vi "相关系数.vi"() -> ()   [LabVIEW 2018]
uses:
  <vilib>/gmath/NI_Gmath.lvlib
panel:
  in  "停止":bool
  out "r^2":dbl format="%.7g"
  out "correlation coefficient r":dbl caption="相关系数r" format="%.7g"
  in  "数组 2":dbl[](array[numeric])
  in  "数组":dbl[](array[numeric])
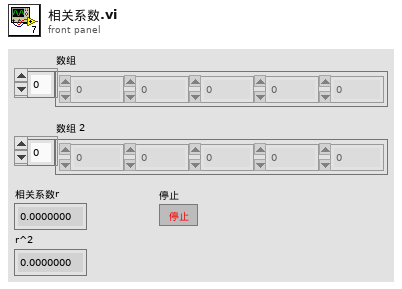
[diagram p1: front panel]
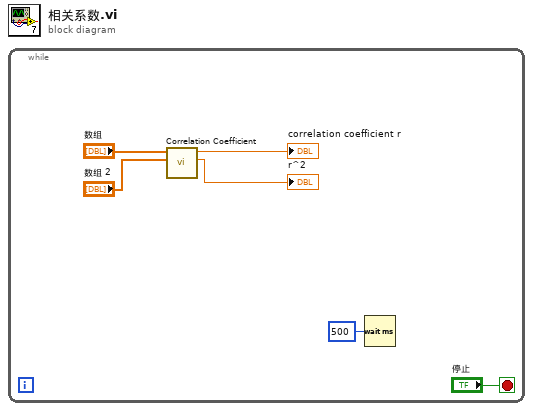
[diagram p0: block diagram]
diagram:
  n1 = while {
    stop <- "停止" stop-if-true
    n2 = call <vilib>:"Correlation Coefficient.vi"("Y"="数组 2", "X"="数组") -> ("r^2"=→"r^2":dbl, "correlation coefficient r"=→"correlation coefficient r":dbl)  [unwired: 8 in]
    n3 = Wait (ms)(milliseconds to wait=u32 500 ("等待时间（毫秒）")) -> ()  [unwired: 1 out]
  }
